vi "Item_NotifyChanged.vi"(8 "error in":errorcluster, 10 "Change Type":T1, 11 "Item Ref":T2) -> (0 "error out":errorcluster)   [LabVIEW 2020, in "FlexWorker_Provider.lvlib"]
uses:
  FlexWorker_Provider.lvlib
  <resource>/Framework/Providers/API/ItemRef.ctl
  <resource>/Framework/Providers/API/mxLvChangeType.ctl
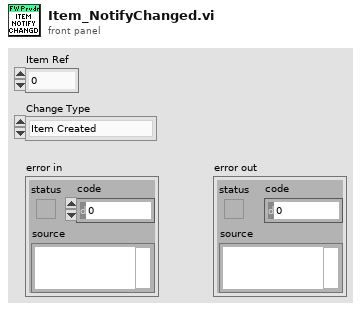
[diagram p1: front panel]
types:
  T1 = typedef "mxLvChangeType.ctl" = enum32{"Item Created", "Item Modified", "File Modified", "File Deleted", "Item Added", "Item Added to SCC", "Item Renamed", "Item Modified For SCC"}
  T2 = typedef "ItemRef.ctl" = u64
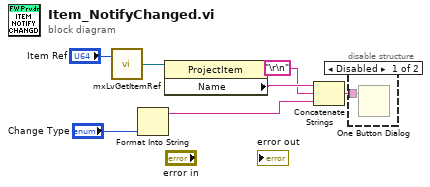
[diagram p0: block diagram]
diagram:
  n1 = call <resource>:"mxLvGetItemRef.vi"("Item"="Item Ref") -> ("Item Refnum"=w6:refnum<vi>)  [unwired: 1 in, 2 out]
  n2 = Format Into String("Change Type") -> (resulting string=w4:string)  [unwired: 3 in, 1 out]
  n3 = property class="ProjectItem"(reference=w6) -> ("Name"=w3:string)  [unwired: 1 in, 2 out]
  n4 = Concatenate Strings(w3, "\r\n", w4) -> (w1:string)
  n5 = disable-structure shown="Disabled" {
    disable-tunnel: w1 -> [w8 _]
    frame Disabled {
      n6 = One Button Dialog(message=w8) -> ()  [unwired: 1 in, 1 out]
    }
    frame Enabled {
    }
  }
